vi "Enqueue Message (All Components).vi"(6 "Priority Message? (F)":bool, 8 "error in (no error)":errorcluster, 9 "Message Data":variant, 10 "Message":string, 11 "Components Message Queues":T1) -> (0 "error out":errorcluster)   [LabVIEW 2019, in "Message Queue.lvlib"]
uses:
  controls/Components Message Queues.ctl
  Message Cluster.ctl
  Enqueue Message (Single).vi
  Message Queue.lvlib
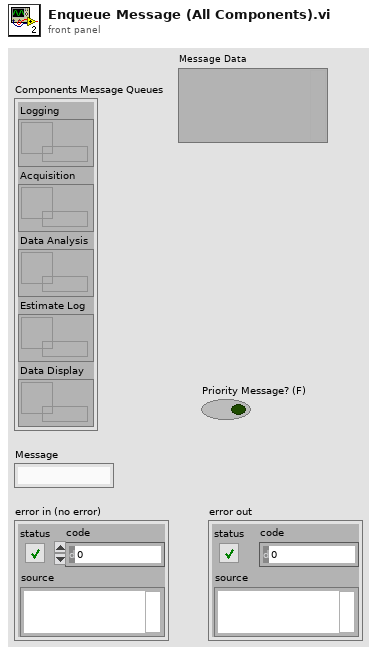
[diagram p1: front panel]
types:
  T1 = typedef "Message Queue.lvlib/Components Message Queues.ctl" = cluster{"Logging":refnum<queue>, "Acquisition":refnum<queue>, "Data Analysis":refnum<queue>, "Estimate Log":refnum<queue>, "Data Display":refnum<queue>}
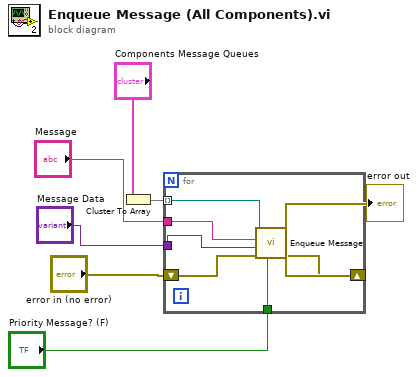
[diagram p0: block diagram]
diagram:
  n1 = Cluster To Array(cluster="Components Message Queues") -> (array=w4:refnum<queue>[])
  n2 = for {
    tunnel: w4 -> [w13] mode=indexing
    tunnel: "Message" -> [w12]
    shift-right: [w10] -> w6
    shift-left: "error in (no error)" -> [w11]
    tunnel: "Message Data" -> [w9]
    tunnel: "Priority Message? (F)" -> [w8]
    n3 = call-poly "Enqueue Message.vi"("Priority Message? (F)"=w8, "error in (no error)"=w11, "Message Data"=w9, "Message"=w12, "Message Queue"=w13) -> ("error out"=w10:errorcluster)  [unwired: 5 in, 1 out]
  }
  "error out" <- w6
